vi "__READ_SP_trace_E4440A.vi"(5 "AVG(0-100)":i32, 6 "wait(s)":dbl, 7 "GPIB":string) -> (0 "error out":errorcluster caption="エラー出力", 3 "data":dbl[](array[numeric]))   [LabVIEW 2017]
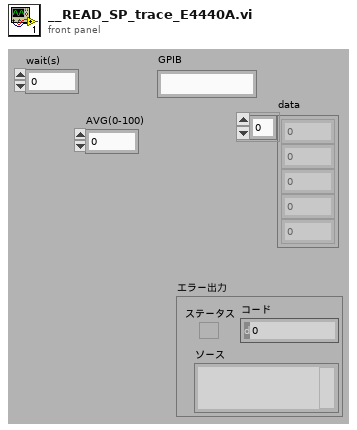
[diagram p1: front panel]
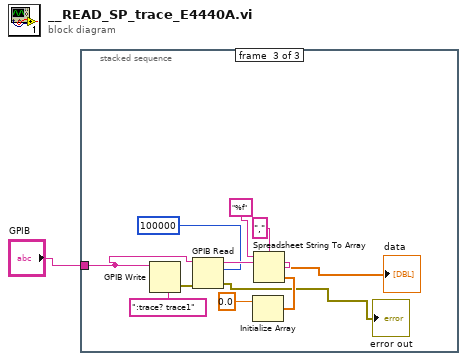
[diagram p0: block diagram]
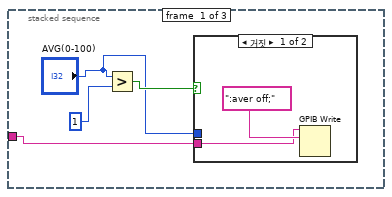
[diagram p2: hidden frame]
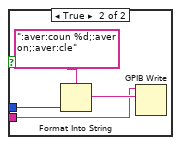
[diagram p3: hidden frame]
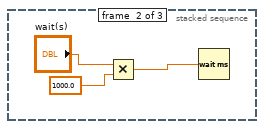
[diagram p4: hidden frame]
diagram:
  n1 = stacked-sequence {
    tunnel: "GPIB" -> [w2 _ w18]
    frame #0 {
      n2 = Greater?(x="AVG(0-100)", y=1) -> (0:w4:bool)
      n3 = case shown="거짓" w4 {
        tunnel: "AVG(0-100)" -> [_ w9]
        tunnel: w2 -> [w6 w8]
        frame False {
          n4 = GPIB Write(0:w6, 1:":aver off;") -> ()  [unwired: 3 in, 2 out]
        }
        frame True {
          n5 = Format Into String(format string=":aver:coun %d;:aver on;:aver:cle", w9) -> (resulting string=w11:string)  [unwired: 2 in, 1 out]
          n6 = GPIB Write(0:w8, 1:w11) -> ()  [unwired: 3 in, 2 out]
        }
      }
    }
    frame #1 {
      n7 = Multiply(x="wait(s)", y=1000.0) -> (x*y=w13:dbl)
      n8 = Wait (ms)(milliseconds to wait=w13) -> ()  [unwired: 1 out]
    }
    frame #2 {
      n9 = GPIB Write(0:w18, 1:":trace? trace1") -> (6:w16:errorcluster)  [unwired: 3 in, 1 out]
      n10 = GPIB Read(0:w18, 1:100000, 3:w16) -> (5:w21:string, 7:→"error out":errorcluster)  [unwired: 2 in, 1 out]
      n11 = Initialize Array(0.0) -> (w24:dbl[])  [unwired: 1 in]
      n12 = Spreadsheet String To Array(delimiter (Tab)=",", format string="%f", spreadsheet string=w21, array type (2D Dbl)=w24) -> (array=→"data":dbl[])
    }
  }
